vi "csm_lumikki_instron_moveToSetpoint_4.vi"(7 "channelInt":i32=1, 8 "rampRate":dbl=1.0, 9 "rampAmplitude":dbl=1.0, 10 "setPointTime":dbl=1.0, 11 "setPoint":dbl=1.0) -> (0 "rampRateOut":dbl, 1 "rampAmplitudeOut":dbl, 2 "setpointTimeOut":dbl, 3 "setpointOut":dbl, 4 "iAmBusyCommandNotExecuted":bool, 5 "channelIntOut":i32)   [LabVIEW 2009]
uses:
  Globals.vi
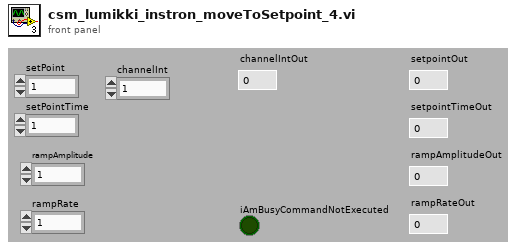
[diagram p1: front panel]
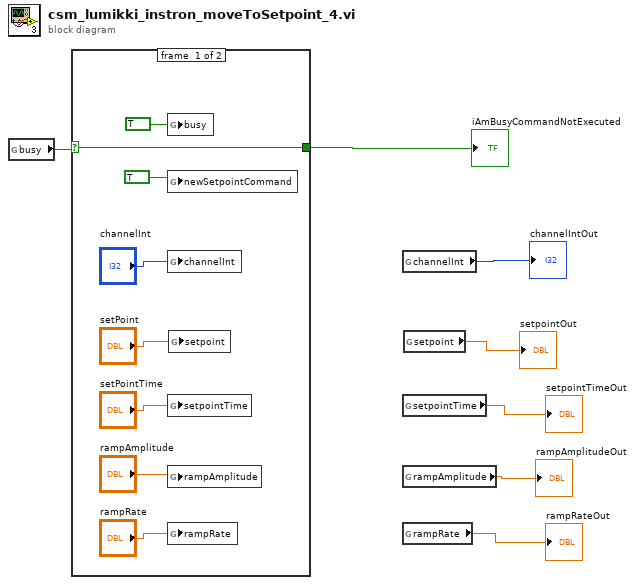
[diagram p0: block diagram]
diagram:
  n1 = global read "Globals.vi" "busy"() -> (w7:bool)
  n2 = case shown="False" w7 {
    selector: w7 -> [w13 w16]
    tunnel: [w13 w16] -> w6
    frame #0 {
      n3 = global write "Globals.vi" "busy"(TRUE ("Busy")) -> ()
      n4 = global write "Globals.vi" "newSetpointCommand"(TRUE ("Busy")) -> ()
      n5 = global write "Globals.vi" "channelInt"("channelInt") -> ()
      n6 = global write "Globals.vi" "setpointTime"("setPointTime") -> ()
      n7 = global write "Globals.vi" "rampAmplitude"("rampAmplitude") -> ()
      n8 = global write "Globals.vi" "rampRate"("rampRate") -> ()
      n9 = global write "Globals.vi" "setpoint"("setPoint") -> ()
    }
    frame #1 {
    }
  }
  "iAmBusyCommandNotExecuted" <- w6
  n10 = global read "Globals.vi" "channelInt"() -> (→"channelIntOut":i32)
  n11 = global read "Globals.vi" "setpointTime"() -> (→"setpointTimeOut":dbl)
  n12 = global read "Globals.vi" "rampAmplitude"() -> (→"rampAmplitudeOut":dbl)
  n13 = global read "Globals.vi" "rampRate"() -> (→"rampRateOut":dbl)
  n14 = global read "Globals.vi" "setpoint"() -> (→"setpointOut":dbl)
